vi "Finish.vi"   [LabVIEW 2018]
doc: "This VI is called just before exiting. It is expected to close I/O refnum, save collected data, etc."
uses:
  <vilib>/Rock Robotics/WPI/Utilities/WPI_GetSetVariantRefNum.vi
types:
  T1 = typedef "WPI_CounterDevRef.ctl" = cluster{"DevStatus":errorcluster, "CntIndex":T2}
  T2 = typedef "FPGA_CounterCtrSystemIndex.ctl" = enum8{"Ctr 0", "Ctr 1", "Ctr 2", "Ctr 3", "Ctr 4", "Ctr 5", "Ctr 6", "Ctr 7", "Invalid"}
  T3 = typedef "WPI_SwitchDevRef.ctl" = cluster{"DevStatus":errorcluster, "DIO Channel":T4, "CntIndex":T2, "Normally Closed":bool}
  T4 = typedef "FPGA_DIOChannel.ctl" = enum8{"DIO 0", "DIO 1", "DIO 2", "DIO 3", "DIO 4", "DIO 5", "DIO 6", "DIO 7", "DIO 8", "DIO 9", "DIO MXP 0", "DIO MXP 1", "DIO MXP 2", "DIO MXP 3", "DIO MXP 4", "DIO MXP 5", "DIO MXP 6", "DIO MXP 7", "DIO MXP 8", "DIO MXP 9", "DIO MXP 10", "DIO MXP 11", "DIO MXP 12", "DIO MXP 13", "DIO MXP 14", "DIO MXP 15", "SPI Port CS1", "SPI Port CS2", "SPI Port CS3", "SPI Port MISO", "SPI Port MOSI", "Invalid"}
  T5 = typedef "WPI_JoystickDevRef.ctl" = cluster{"Device":T6}
  T6 = typedef "WPI_JoystickDeviceEnum.ctl" = enum16{"USB 0", "USB 1", "USB 2", "USB 3", "USB 4", "USB 5"}
  T7 = typedef "WPI_RobotDriveDevRef.ctl" = cluster{"DevStatus":errorcluster, "Motors[]":T8[], "Square Inputs":bool, "Max Output":dbl}
  T8 = typedef "WPI_MotorControlDeviceRef.ctl" = cluster{"DeviceStatus":errorcluster, "Type":T9, "PWM":cluster{"PWM Channel":T10, "DeadBand":T11}, "CAN":cluster{"Device Number":u8, "SetOutput VI Ref":variant, "GetOutput VI Ref":variant, "Enable VI Ref":variant, "Disable VI Ref":variant, "Data":variant}, "Invert":bool, "DIO PWM":cluster{"PWM \"Enable\" Channel":T10, "DIOChannel":T4, "PWM Rate":dbl}}
  T9 = typedef "WPI_MotorControlType.ctl" = enum16{"PWM", "CAN", "DIO PWM"}
  T10 = typedef "FPGA_DIOPWMChannel.ctl" = enum8{"PWM 0", "PWM 1", "PWM 2", "PWM 3", "PWM 4", "PWM 5", "PWM 6", "PWM 7", "PWM 8", "PWM 9", "PWM MXP 0", "PWM MXP 1", "PWM MXP 2", "PWM MXP 3", "PWM MXP 4", "PWM MXP 5", "PWM MXP 6", "PWM MXP 7", "PWM MXP 8", "PWM MXP 9", "Invalid"}
  T11 = typedef "WPI_PWMDeadband.ctl" = cluster{"Name":string, "maxPositivePwm":i32, "minPositivePwm":i32, "centerPwm":i32, "maxNegativePwm":i32, "minNegativePwm":i32, "angularRange":u16}
  T12 = typedef "WPI_SolenoidDevRef.ctl" = cluster{"DevStatus":errorcluster, "Pneumatics Control Module":u8, "Forward Solenoid Channel":T13, "Reverse Solenoid Channel":T13}
  T13 = typedef "WPI_SolenoidChannel.ctl" = enum8{"Solenoid 0", "Solenoid 1", "Solenoid 2", "Solenoid 3", "Solenoid 4", "Solenoid 5", "Solenoid 6", "Solenoid 7", "Invalid"}
  T14 = typedef "WPI_EncoderDevRef.ctl" = cluster{"DevStatus":errorcluster, "EncoderIndex":T15, "CounterIndex":T2, "DistancePerCount":dbl, "Decoding Type":T16}
  T15 = typedef "FPGA_EncoderIdx.ctl" = enum8{"Enc 0", "Enc 1", "Enc 2", "Enc 3", "Enc 4", "Enc 5", "Enc 6", "Enc 7", "Invalid"}
  T16 = typedef "WPI_EncoderType.ctl" = enum16{"1x", "2x", "4x"}
  T17 = typedef "WPI_CompressorDevRef.ctl" = cluster{"DevStatus":errorcluster, "Pneumatics Control Module":u8}
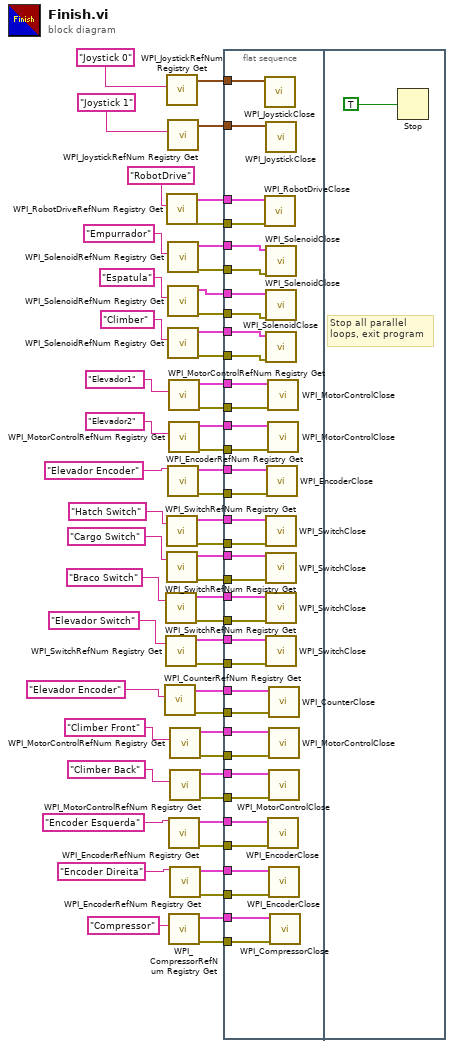
[diagram p0: block diagram]
diagram:
  n1 = call <vilib>:"WPI_CounterRefNum Registry Get.vi"("refnum name"="Elevador Encoder") -> ("error out"=w17:errorcluster, "CounterDevRef"=w18:T1)  [unwired: 9 in]
  n2 = call <vilib>:"WPI_SwitchRefNum Registry Get.vi"("refnum name"="Braco Switch") -> ("error out"=w23:errorcluster, "SwitchDevRef"=w24:T3)  [unwired: 9 in]
  n3 = call <vilib>:"WPI_SwitchRefNum Registry Get.vi"("refnum name"="Elevador Switch") -> ("error out"=w21:errorcluster, "SwitchDevRef"=w22:T3)  [unwired: 9 in]
  n4 = call <vilib>:"WPI_JoystickRefNum Registry Get.vi"("refnum name"="Joystick 0") -> ("JoystickDevRef"=w47:T5)  [unwired: 1 in, 9 out]
  n5 = call <vilib>:"WPI_RobotDriveRefNum Registry Get.vi"("refnum name"="RobotDrive") -> ("error out"=w44:errorcluster, "RobotDriveDevRef"=w45:T7)  [unwired: 1 in, 8 out]
  n6 = call <vilib>:"WPI_SwitchRefNum Registry Get.vi"("refnum name"="Hatch Switch") -> ("error out"=w25:errorcluster, "SwitchDevRef"=w26:T3)  [unwired: 9 in]
  n7 = call <vilib>:"WPI_SwitchRefNum Registry Get.vi"("refnum name"="Cargo Switch") -> ("error out"=w19:errorcluster, "SwitchDevRef"=w20:T3)  [unwired: 9 in]
  n8 = call <vilib>:"WPI_JoystickRefNum Registry Get.vi"("refnum name"="Joystick 1") -> ("JoystickDevRef"=w46:T5)  [unwired: 1 in, 9 out]
  n9 = call <vilib>:"WPI_SolenoidRefNum Registry Get.vi"("refnum name"="Empurrador") -> ("error out"=w42:errorcluster, "SolenoidDevRef"=w43:T12)  [unwired: 9 in]
  n10 = call <vilib>:"WPI_SolenoidRefNum Registry Get.vi"("refnum name"="Espatula") -> ("error out"=w40:errorcluster, "SolenoidDevRef"=w41:T12)  [unwired: 9 in]
  n11 = call <vilib>:"WPI_SolenoidRefNum Registry Get.vi"("refnum name"="Climber") -> ("error out"=w38:errorcluster, "SolenoidDevRef"=w39:T12)  [unwired: 9 in]
  n12 = call <vilib>:"WPI_EncoderRefNum Registry Get.vi"("refnum name"="Elevador Encoder") -> ("error out"=w31:errorcluster, "EncoderDevRef"=w32:T14)  [unwired: 9 in]
  n13 = call <vilib>:"WPI_MotorControlRefNum Registry Get.vi"("refnum name"="Elevador1") -> ("error out"=w36:errorcluster, "MotorControlDevRef"=w37:T8)  [unwired: 9 in]
  n14 = call <vilib>:"WPI_MotorControlRefNum Registry Get.vi"("refnum name"="Elevador2") -> ("error out"=w34:errorcluster, "MotorControlDevRef"=w35:T8)  [unwired: 9 in]
  n15 = call <vilib>:"WPI_EncoderRefNum Registry Get.vi"("refnum name"="Encoder Esquerda") -> ("error out"=w9:errorcluster, "EncoderDevRef"=w8:T14)  [unwired: 9 in]
  n16 = call <vilib>:"WPI_CompressorRefNum Registry Get.vi"("refnum name"="Compressor") -> ("error out"=w2:errorcluster, "CompressorDevRef"=w3:T17)  [unwired: 9 in]
  n17 = call <vilib>:"WPI_MotorControlRefNum Registry Get.vi"("refnum name"="Climber Front") -> ("error out"=w13:errorcluster, "MotorControlDevRef"=w12:T8)  [unwired: 9 in]
  n18 = call <vilib>:"WPI_MotorControlRefNum Registry Get.vi"("refnum name"="Climber Back") -> ("error out"=w15:errorcluster, "MotorControlDevRef"=w14:T8)  [unwired: 9 in]
  n19 = call <vilib>:"WPI_EncoderRefNum Registry Get.vi"("refnum name"="Encoder Direita") -> ("error out"=w4:errorcluster, "EncoderDevRef"=w5:T14)  [unwired: 9 in]
  n20 = flat-sequence {
    tunnel: w47 -> [w91]
    tunnel: w46 -> [w90]
    tunnel: w45 -> [w89]
    tunnel: w44 -> [w88]
    tunnel: w43 -> [w87]
    tunnel: w42 -> [w86]
    tunnel: w41 -> [w85]
    tunnel: w40 -> [w84]
    tunnel: w39 -> [w83]
    tunnel: w38 -> [w82]
    tunnel: w37 -> [w81]
    tunnel: w36 -> [w80]
    tunnel: w35 -> [w79]
    tunnel: w34 -> [w78]
    tunnel: w32 -> [w77]
    tunnel: w31 -> [w76]
    tunnel: w26 -> [w75]
    tunnel: w25 -> [w74]
    tunnel: w24 -> [w73]
    tunnel: w23 -> [w72]
    tunnel: w22 -> [w71]
    tunnel: w21 -> [w70]
    tunnel: w20 -> [w69]
    tunnel: w19 -> [w68]
    tunnel: w18 -> [w67]
    tunnel: w17 -> [w66]
    tunnel: w12 -> [w62]
    tunnel: w13 -> [w63]
    tunnel: w14 -> [w64]
    tunnel: w15 -> [w65]
    tunnel: w8 -> [w60]
    tunnel: w9 -> [w61]
    tunnel: w5 -> [w59]
    tunnel: w4 -> [w58]
    tunnel: w3 -> [w57]
    tunnel: w2 -> [w56]
    frame #0 {
      n21 = call <vilib>:"WPI_JoystickClose.vi"("JoystickDevRef"=w91) -> ()  [unwired: 11 out]
      n22 = call <vilib>:"WPI_RobotDriveClose.vi"("error in (no error)"=w88, "RobotDriveDevRef"=w89) -> ()  [unwired: 10 out]
      n23 = call <vilib>:"WPI_JoystickClose.vi"("JoystickDevRef"=w90) -> ()  [unwired: 11 out]
      n24 = call <vilib>:"WPI_SolenoidClose.vi"("error in (no error)"=w86, "SolenoidDevRef"=w87) -> ()  [unwired: 9 in, 1 out]
      n25 = call <vilib>:"WPI_SolenoidClose.vi"("error in (no error)"=w84, "SolenoidDevRef"=w85) -> ()  [unwired: 9 in, 1 out]
      n26 = call <vilib>:"WPI_SolenoidClose.vi"("error in (no error)"=w82, "SolenoidDevRef"=w83) -> ()  [unwired: 9 in, 1 out]
      n27 = call <vilib>:"WPI_SwitchClose.vi"("error in (no error)"=w74, "SwitchDevRef"=w75) -> ()  [unwired: 9 in, 1 out]
      n28 = call <vilib>:"WPI_SwitchClose.vi"("error in (no error)"=w68, "SwitchDevRef"=w69) -> ()  [unwired: 9 in, 1 out]
      n29 = call <vilib>:"WPI_SwitchClose.vi"("error in (no error)"=w72, "SwitchDevRef"=w73) -> ()  [unwired: 9 in, 1 out]
      n30 = call <vilib>:"WPI_SwitchClose.vi"("error in (no error)"=w70, "SwitchDevRef"=w71) -> ()  [unwired: 9 in, 1 out]
      n31 = call <vilib>:"WPI_EncoderClose.vi"("error in (no error)"=w76, "EncoderDevRef"=w77) -> ()  [unwired: 9 in, 1 out]
      n32 = call <vilib>:"WPI_MotorControlClose.vi"("error in"=w80, "MotorControlDevRef"=w81) -> ()  [unwired: 9 in, 1 out]
      n33 = call <vilib>:"WPI_MotorControlClose.vi"("error in"=w78, "MotorControlDevRef"=w79) -> ()  [unwired: 9 in, 1 out]
      n34 = call <vilib>:"WPI_EncoderClose.vi"("error in (no error)"=w61, "EncoderDevRef"=w60) -> ()  [unwired: 9 in, 1 out]
      n35 = call <vilib>:"WPI_CounterClose.vi"("error in (no error)"=w66, "CounterDevRef"=w67) -> ()  [unwired: 9 in, 1 out]
      n36 = call <vilib>:"WPI_MotorControlClose.vi"("error in"=w63, "MotorControlDevRef"=w62) -> ()  [unwired: 9 in, 1 out]
      n37 = call <vilib>:"WPI_MotorControlClose.vi"("error in"=w65, "MotorControlDevRef"=w64) -> ()  [unwired: 9 in, 1 out]
      n38 = call <vilib>:"WPI_EncoderClose.vi"("error in (no error)"=w58, "EncoderDevRef"=w59) -> ()  [unwired: 9 in, 1 out]
      n39 = call <vilib>:"WPI_CompressorClose.vi"("error in (no error)"=w56, "CompressorDevRef"=w57) -> ()  [unwired: 9 in, 1 out]
    }
    frame #1 {
      # "Stop all parallel\nloops, exit program"
      n40 = Stop(stop? (T)=TRUE ("Quit")) -> ()
    }
  }
